vi "tool_Unicode_Display String Arrray (2D) Text.vi"(5 "Interpret as Unicode (T)":bool, 6 "error in":errorcluster, 8 "Value":string[][](array[string]), 9 "String Array (2D) Ref":refnum<vi>) -> (0 "error out":errorcluster, 3 "String Array (2D) Ref":refnum<vi>)   [LabVIEW 2009]
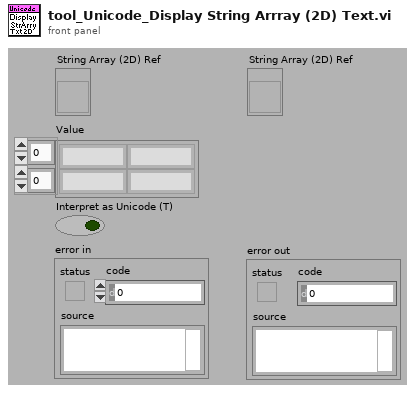
[diagram p1: front panel]
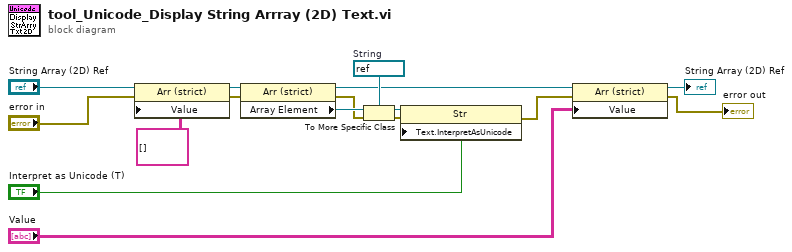
[diagram p0: block diagram]
diagram:
  w14 = refnum<vi> refnum  # String
  n1 = property class="Arr (strict)"(reference="String Array (2D) Ref", error in="error in", "Value"=string[][] []) -> (reference out=w9:refnum<vi>, error out=w8:errorcluster)
  n2 = property class="Arr (strict)"(reference=w9, error in=w8) -> (reference out=w10:refnum<vi>, error out=w13:errorcluster, "Array Element"=w16:refnum<vi>)
  n3 = To More Specific Class(target class=w14, reference=w16, error in=w13) -> (specific class reference=w15:refnum<vi>, error out=w12:errorcluster)
  n4 = property class="Str"(reference=w15, error in=w12, "Text.InterpretAsUnicode"="Interpret as Unicode (T)") -> (error out=w11:errorcluster)  [unwired: 1 out]
  n5 = property class="Arr (strict)"(reference=w10, error in=w11, "Value"="Value") -> (reference out=→"String Array (2D) Ref":refnum<vi>, error out=→"error out":errorcluster)
